vi "Camera.vi"(0 "Camera in":refnum<class "Camera.lvclass">, 1 "Stop":bool, 4 "BCG Image Processing":T3={"Brightness"=128.0, "Contrast"=45.0, "Gamma"=1.0} {"Brightness" scale=0.0..400.0; "Contrast" scale=0.0..90.0; "Gamma" scale=0.005..5.0}, 5 "error in (no error)":errorcluster, 6 "Machine Vision":T5, 7 "Camera settings":T2={"Gamma"=1.0, "Gain"=7, "Sharpness"=0, "Contrast"=0.009999999999999995, "Exposure"=0.0004073180282999787} {"Exposure" min=0.000244140625 max=0.5 scale=0.0002..0.5; "Contrast" min=0.0 max=1.0 scale=0.001..1.0; "Sharpness" min=0 max=2 step=1 scale=0.0..2.0; "Gain" min=0 max=100 step=1 scale=0.1..100.0; "Gamma" min=0.01 max=10.0 scale=0.01..10.0}, 10 "Material":T4, 12 "Loop 0":bool, 13 "Override presets":bool) -> (11 "Radius (Real-World)":dbl, 14 "Camera out":refnum<class "Camera.lvclass">, 15 "Average Strength":dbl, 16 "Global Report":T1 {"Mean Value" format="%.2f"; "%" format="%.2f"; "Area (calibrated)" format="%.2f"; "Maximal Value" format="%.2f"; "Minimal Value" format="%.2f"; "Standard Variation" format="%.2f"}, 17 "Image":T6(plugin-control), 18 "Camera":dbl[](array[numeric]), 19 "error out":errorcluster)   [LabVIEW 2021, in "Camera.lvclass"]
uses:
  Camera.lvclass
  Machine Vision.ctl
  Material.ctl
  Image processing.ctl
  Camera settings.ctl
  <vilib>/vision/NI_Vision_Development_Module.lvlib
panel:
  out "Y":sgl
  out "X":sgl
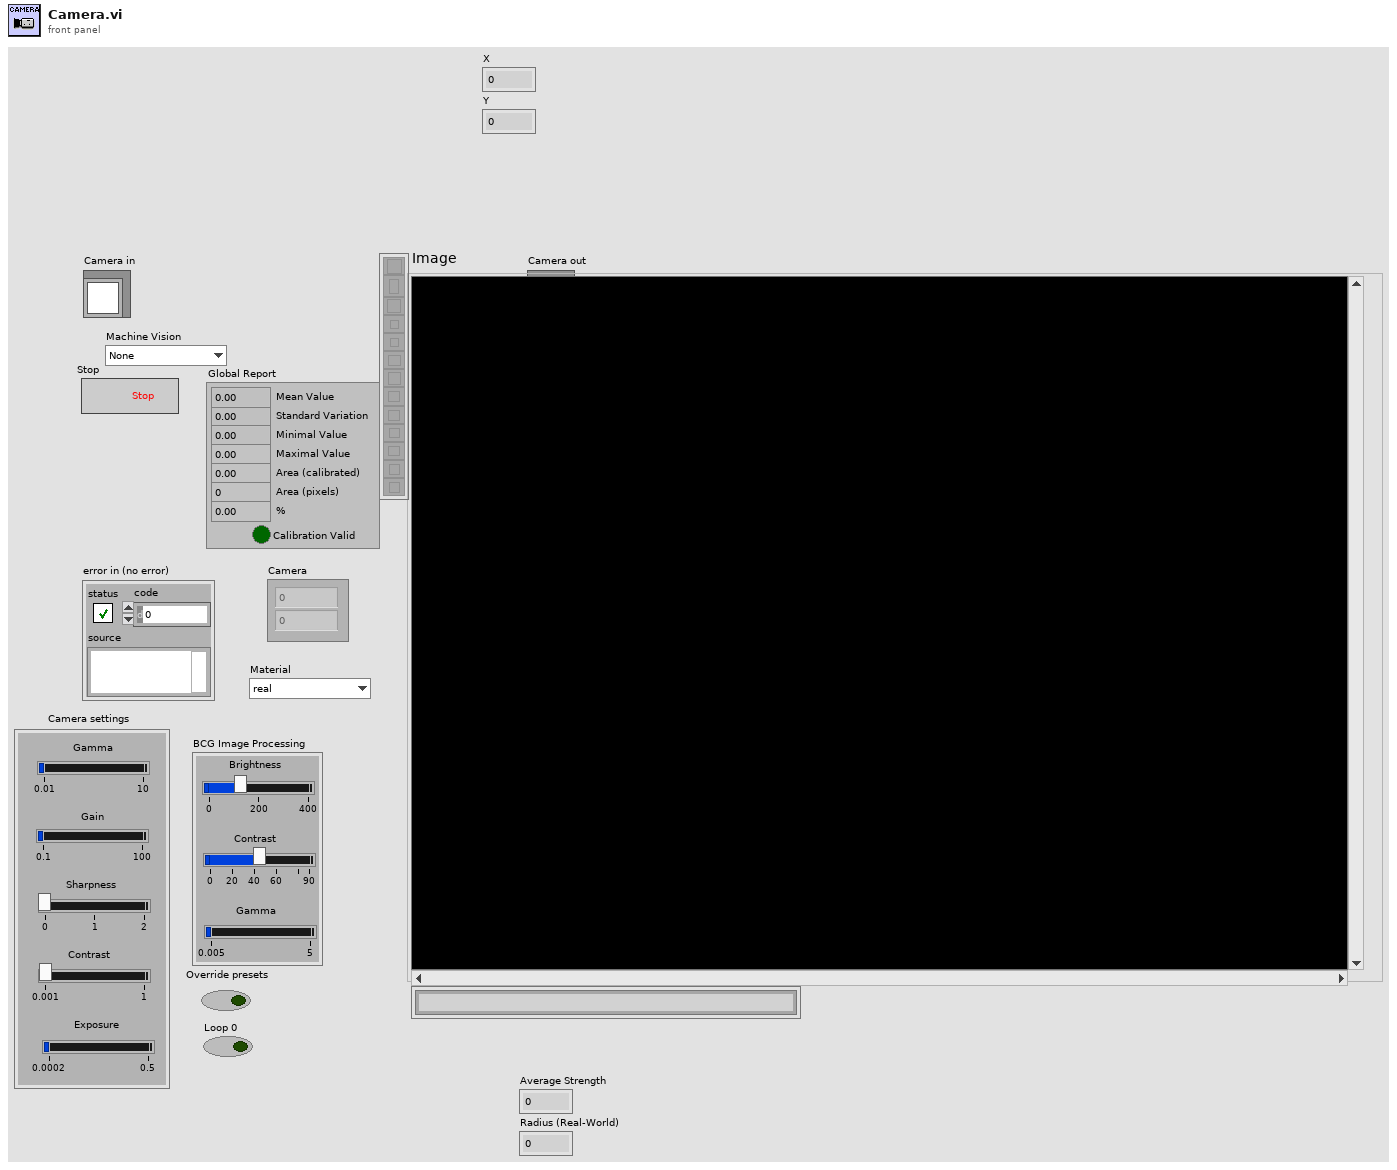
[diagram p1: front panel]
types:
  T1 = cluster{"Mean Value":sgl, "Standard Variation":sgl, "Minimal Value":sgl, "Maximal Value":sgl, "Area (calibrated)":sgl, "Area (pixels)":u32, "%":sgl, "Calibration Valid":bool}
  T2 = typedef "Camera.lvclass/Camera settings.ctl" = cluster{"Gamma":dbl, "Gain":i64, "Sharpness":i64, "Contrast":dbl, "Exposure":dbl}
  T3 = typedef "Camera.lvclass/Image processing.ctl" = cluster{"Brightness":sgl, "Contrast":sgl, "Gamma":sgl}
  T4 = typedef "Camera.lvclass/Material.ctl" = enum16{"real", "dummy", "PETG"}
  T5 = typedef "Camera.lvclass/Machine Vision.ctl" = enum16{"None", "Tray Fiducials", "Sensor Fiducials", "HPK Silicon", "Partial Hexaboard", "Partial Hexaboard Test", "100um dot", "Hexaboard", "Corner (TL, BR)", "Corner (BL, TR)", "V3 Sensor Cross", "V3 Sensor Circle"}
  T6 = typedef "IMAQ Image.ctl" = refnum<image>
  T7 = cluster{"Center (Pixels)":cluster{"X":sgl, "Y":sgl}, "Radius (Pixels)":dbl, "Center (Real-World)":cluster{"X":sgl, "Y":sgl}, "Radius (Real-World)":dbl, "Roundness (Real-World)":dbl, "Average Strength":dbl, "Average SNR (dB)":dbl}
  T8 = typedef "Edge New.ctl" = cluster{"Location (Pixel)":cluster{"X":sgl, "Y":sgl}, "Location (Real-World)":cluster{"X":sgl, "Y":sgl}, "Distance (Pixel)":dbl, "Distance (Real-World)":dbl, "Strength":dbl, "Noise":dbl, "Rising?":bool}
  T9 = cluster{"output string":sgl, "output string":sgl}
  T10 = typedef "ROI Descriptor" = cluster{"Global Rectangle":i32[], "Contours":cluster{"ID":enum32{"External", "Internal"}, "Type":u32, "Coordinates":i32[]}[]}
  T11 = typedef "Image Type" = u32
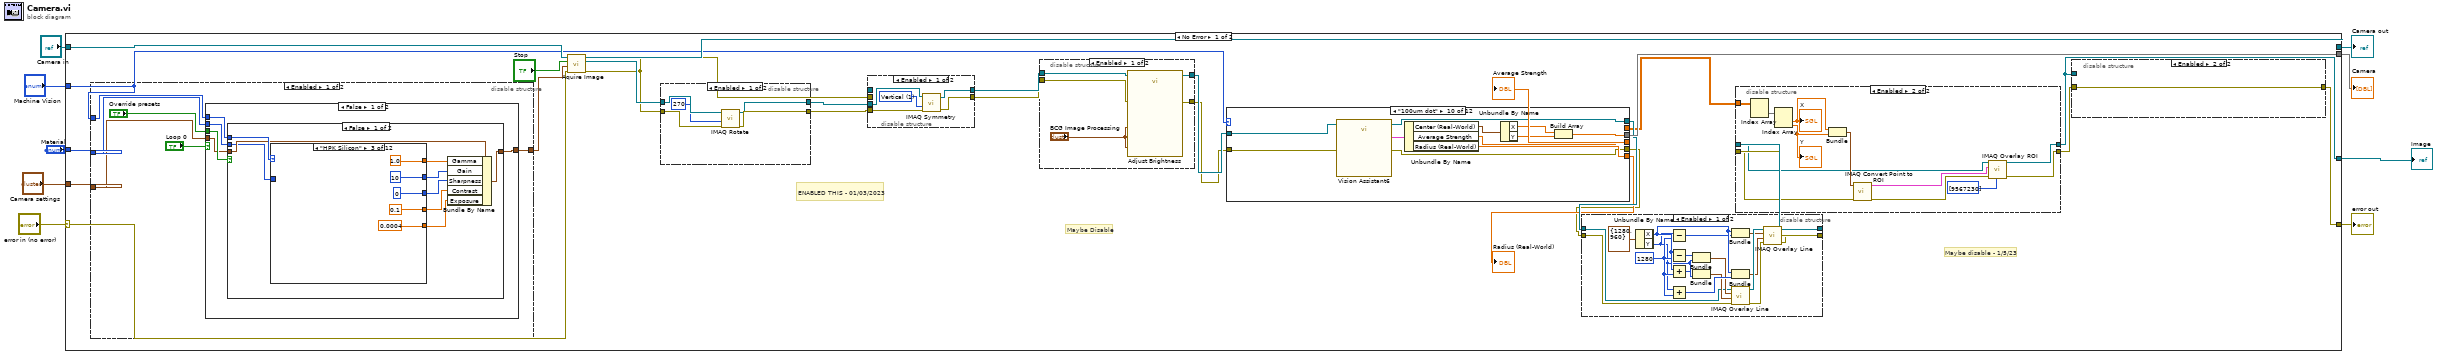
[diagram p0: block diagram]
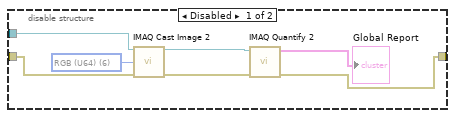
[diagram p2: hidden frame]
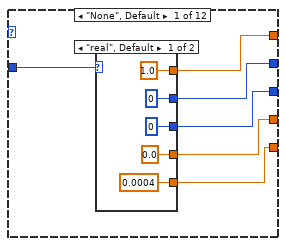
[diagram p7: hidden frame]
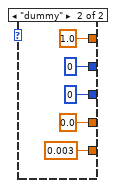
[diagram p8: hidden frame]
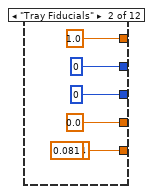
[diagram p9: hidden frame]
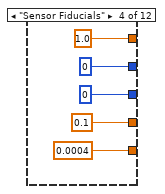
[diagram p10: hidden frame]
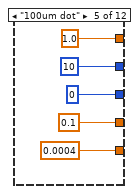
[diagram p11: hidden frame]
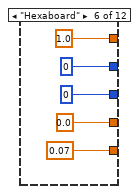
[diagram p12: hidden frame]
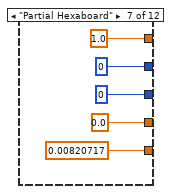
[diagram p13: hidden frame]
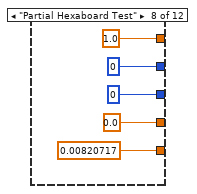
[diagram p14: hidden frame]
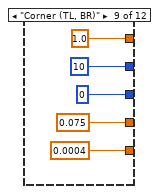
[diagram p15: hidden frame]
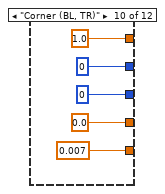
[diagram p16: hidden frame]
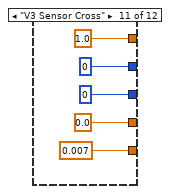
[diagram p17: hidden frame]
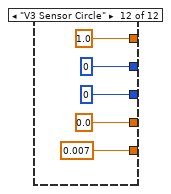
[diagram p18: hidden frame]
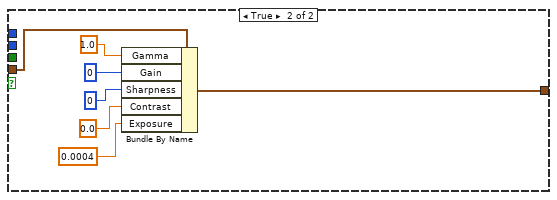
[diagram p20: hidden frame]
diagram:
  n1 = case shown="No Error" "error in (no error)" {
    selector: "error in (no error)" -> [w20 w327]
    tunnel: [w10 w327] -> w8
    tunnel: [w34 w326] -> w7
    tunnel: "Camera in" -> [w35 w326]
    tunnel: [w33 _] -> w5
    tunnel: [w12 _] -> w4
    tunnel: "Machine Vision" -> [w29 _]
    tunnel: "Camera settings" -> [w30 _]
    tunnel: "Material" -> [w28 _]
    frame No Error {
      # "Maybe Disable"
      # "Maybe disable - 1/5/23"
      # "ENABLED THIS - 01/03/2023"
      n2 = disable-structure shown="Enabled" {
        disable-tunnel: w29 -> [w98 _]
        disable-tunnel: w30 -> [w97 w192]
        disable-tunnel: [w96 w192] -> w31
        disable-tunnel: w28 -> [w93 _]
        frame Enabled {
          n3 = case shown="False" "Loop 0" {
            tunnel: "Override presets" -> [w103 _]
            tunnel: w98 -> [w102 _]
            tunnel: w97 -> [w101 w191]
            tunnel: [w100 w190] -> w96
            tunnel: w93 -> [w99 _]
            frame False {
              n4 = case shown="False" w103 {
                tunnel: w102 -> [w112 _]
                tunnel: w101 -> [w111 w184]
                tunnel: [w105 w184] -> w100
                tunnel: w99 -> [w104 _]
                frame False {
                  n5 = case shown="\"HPK Silicon\"" w112 {
                    tunnel: [w117 1.0 ("Gamma::Value") 1.0 ("Gamma::Value") 1.0 ("Gamma::Value") 1.0 ("Gamma::Value") 1.0 ("Gamma::Value") 1.0 ("Gamma::Value") 1.0 ("Gamma::Value") 1.0 ("Gamma::Value") 1.0 ("Gamma::Value") 1.0 ("Gamma::Value") 1.0 ("Gamma::Value")] -> w110
                    tunnel: [w113 i64 0 ("Gain::Value") i64 10 ("Gain::Value") i64 0 ("Gain::Value") i64 10 ("Gain::Value") i64 0 ("Gain::Value") i64 0 ("Gain::Value") i64 0 ("Gain::Value") i64 10 ("Gain::Value") i64 0 ("Gain::Value") i64 0 ("Gain::Value") i64 0 ("Gain::Value")] -> w109
                    tunnel: [w114 i64 0 ("Sharpness::Value") i64 0 ("Sharpness::Value") i64 0 ("Sharpness::Value") i64 0 ("Sharpness::Value") i64 0 ("Sharpness::Value") i64 0 ("Sharpness::Value") i64 0 ("Sharpness::Value") i64 0 ("Sharpness::Value") i64 0 ("Sharpness::Value") i64 0 ("Sharpness::Value") i64 0 ("Sharpness::Value")] -> w108
                    tunnel: [w115 0.0 ("Contrast::Value") 0.1 ("Contrast::Value") 0.1 ("Contrast::Value") 0.1 ("Contrast::Value") 0.0 ("Contrast::Value") 0.0 ("Contrast::Value") 0.0 ("Contrast::Value") 0.075 ("Contrast::Value") 0.0 ("Contrast::Value") 0.0 ("Contrast::Value") 0.0 ("Contrast::Value")] -> w107
                    tunnel: [w116 0.081 ("Exposure::Value") 0.0004 ("Exposure::Value") 0.0004 ("Exposure::Value") 0.0004 ("Exposure::Value") 0.07 ("Exposure::Value") 0.00820717 ("Exposure::Value") 0.00820717 ("Exposure::Value") 0.0004 ("Exposure::Value") 0.007 ("Exposure::Value") 0.007 ("Exposure::Value") 0.007 ("Exposure::Value")] -> w106
                    tunnel: w104 -> [w118 _ _ _ _ _ _ _ _ _ _ _]
                    frame "None", Default {
                      n6 = case shown="\"real\", Default" w118 {
                        tunnel: [1.0 ("Gamma::Value") 1.0 ("Gamma::Value")] -> w117
                        tunnel: [0.0004 ("Exposure::Value") 0.003 ("Exposure::Value")] -> w116
                        tunnel: [0.0 ("Contrast::Value") 0.0 ("Contrast::Value")] -> w115
                        tunnel: [i64 0 ("Sharpness::Value") i64 0 ("Sharpness::Value")] -> w114
                        tunnel: [i64 0 ("Gain::Value") i64 0 ("Gain::Value")] -> w113
                        frame "real", Default {
                        }
                        frame "dummy" {
                        }
                      }
                    }
                    frame "Tray Fiducials" {
                      (unwired) 0.0004 ("Exposure::Value")
                    }
                    frame "HPK Silicon" {
                    }
                    frame "Sensor Fiducials" {
                    }
                    frame "100um dot" {
                    }
                    frame "Hexaboard" {
                    }
                    frame "Partial Hexaboard" {
                    }
                    frame "Partial Hexaboard Test" {
                    }
                    frame "Corner (TL, BR)" {
                    }
                    frame "Corner (BL, TR)" {
                    }
                    frame "V3 Sensor Cross" {
                    }
                    frame "V3 Sensor Circle" {
                    }
                  }
                  n7 = Bundle By Name(cluster=w111, "Gamma"=w110, "Gain"=w109, "Sharpness"=w108, "Contrast"=w107, "Exposure"=w106) -> (w105:T2)
                }
                frame True {
                }
              }
            }
            frame True {
              n8 = Bundle By Name(cluster=w191, "Gamma"=1.0, "Gain"=i64 0, "Sharpness"=i64 0, "Contrast"=0.0, "Exposure"=0.0004) -> (w190:T2)
            }
          }
        }
        frame Disabled {
        }
      }
      n9 = call-dynamic "Aquire Image.vi"("error in (no error)"=w20, "Cluster"=w31, "Stop"="Stop", "Camera in"=w35) -> ("error out"=w19:errorcluster, "Image Out"=w32:T6, "Camera out"=w34:refnum<class "Camera.lvclass">)  [unwired: 5 in]
      n10 = disable-structure shown="Enabled" {
        disable-tunnel: w32 -> [w49 w51]
        disable-tunnel: w19 -> [w48 w50]
        disable-tunnel: [w46 w50] -> w14
        disable-tunnel: [w45 w51] -> w13
        frame Enabled {
          n11 = call "IMAQ Rotate"("error in (no error)"=w48, "Angle (degrees)"=270, "Image Src"=w49) -> ("error out"=w46:errorcluster, "Image Dst Out"=w45:T6)  [unwired: 7 in]
        }
        frame Disabled {
        }
      }
      n12 = disable-structure shown="Enabled" {
        disable-tunnel: _ -> [_ w199]
        disable-tunnel: [w197 w199] -> w27
        disable-tunnel: w19 -> [_ w198]
        disable-tunnel: [w195 w198] -> w18
        disable-tunnel: w14 -> [w194 _]
        disable-tunnel: w13 -> [w193 _]
        frame Enabled {
          w196 = u32 1 items=["Horizontal", "Vertical", "Central", "1st Diagonal", "2nd Diagonal"] ("Type of Symmetry")
          n13 = call "IMAQ Symmetry"("error in (no error)"=w194, "Type of Symmetry"=w196, "Image Src"=w193) -> ("error out"=w195:errorcluster, "Image Dst Out"=w197:T6)  [unwired: 2 in]
        }
        frame Disabled {
        }
      }
      n14 = disable-structure shown="Enabled" {
        disable-tunnel: w27 -> [w90 w91]
        disable-tunnel: [w88 w91] -> w26
        disable-tunnel: w18 -> [w87 w92]
        disable-tunnel: [w86 w92] -> w17
        frame Enabled {
          n15 = call "Adjust Brightness"("Image In"=w90, "Red BCG Values (Brightness 1)"="BCG Image Processing", "Green BCG Values (Brightness 1)"="BCG Image Processing", "Blue BCG Values (Brightness 1)"="BCG Image Processing", "error in"=w87) -> ("Image Out"=w88:T6, "error out"=w86:errorcluster)  [unwired: 21 in]
        }
        frame Disabled {
        }
      }
      n16 = case shown="\"100um dot\"" w29 {
        tunnel: [w204 w214 w222 w233 w244 w255 w266 w275 w286 w297 w303 w315] -> w33
        tunnel: [w206 w216 w223 w234 w245 w256 w268 w276 w287 w298 w307 w319] -> w25
        tunnel: w26 -> [w207 w216 w221 w232 w243 w254 w265 w273 w284 w295 w308 w320]
        tunnel: [w202 0.0 ("Radius (Real-World)") w219 w230 w241 w252 0.0 ("Radius (Real-World)") w272 w283 w294 0.0 ("Radius (Real-World)") 0.0 ("Radius (Real-World)")] -> w23
        tunnel: [w203 0.0 ("Strength") w220 w231 w242 w253 _ w271 w282 w293 w313 w325] -> w22
        tunnel: [_ _ _ _ _ _ w264 _ _ _ _ _] -> w21
        tunnel: w17 -> [w201 w215 w217 w228 w239 w250 w263 w270 w281 w292 w306 w318]
        tunnel: [w200 w215 w218 w229 w240 w251 w262 w269 w280 w291 w305 w317] -> w16
        frame "Tray Fiducials", Default {
          n17 = call "Vision Assistant"("Image In"=w207, "error in"=w201) -> ("Image Out"=w206:T6, "Fitted Circle (Find Circular Edge 1)"=w205:T7, "error out"=w200:errorcluster)  [unwired: 23 in]
          n18 = Unbundle By Name(w205) -> ("Center (Real-World)"=w208:cluster{"X":sgl, "Y":sgl}, "Average Strength"=w203:dbl, "Radius (Real-World)"=w202:dbl)
          n19 = Unbundle By Name(w208) -> ("X"=w210:sgl, "Y"=w209:sgl)
          n20 = Build Array(w210, w209) -> (w204:sgl[])
        }
        frame "None" {
          n21 = Initialize Array(0.0 ("element")) -> (w214:dbl[])  [unwired: 1 in]
        }
        frame "Hexaboard" {
          n22 = call "Vision Assistant2"("Image In"=w221, "error in"=w217) -> ("Image Out"=w223:T6, "Fitted Circle (Find Circular Edge 1)"=w225:T7, "error out"=w218:errorcluster)  [unwired: 23 in]
          n23 = Unbundle By Name(w225) -> ("Center (Real-World)"=w227:cluster{"X":sgl, "Y":sgl}, "Average Strength"=w220:dbl, "Radius (Real-World)"=w219:dbl)
          n24 = Unbundle By Name(w227) -> ("X"=w226:sgl, "Y"=w224:sgl)
          n25 = Build Array(w226, w224) -> (w222:sgl[])
        }
        frame "V3 Sensor Circle" {
          n26 = call "Vision Assistant4"("Image In"=w232, "error in"=w228) -> ("Image Out"=w234:T6, "Fitted Circle (Find Circular Edge 1)"=w236:T7, "error out"=w229:errorcluster)  [unwired: 23 in]
          n27 = Unbundle By Name(w236) -> ("Center (Real-World)"=w238:cluster{"X":sgl, "Y":sgl}, "Average Strength"=w231:dbl, "Radius (Real-World)"=w230:dbl)
          n28 = Unbundle By Name(w238) -> ("X"=w237:sgl, "Y"=w235:sgl)
          n29 = Build Array(w237, w235) -> (w233:sgl[])
        }
        frame "Partial Hexaboard" {
          n30 = call "Vision Assistant20"("Image In"=w243, "error in"=w239) -> ("Image Out"=w245:T6, "Fitted Circle (Find Circular Edge 1)"=w247:T7, "error out"=w240:errorcluster)  [unwired: 23 in]
          n31 = Unbundle By Name(w247) -> ("Center (Real-World)"=w249:cluster{"X":sgl, "Y":sgl}, "Average Strength"=w242:dbl, "Radius (Real-World)"=w241:dbl)
          n32 = Unbundle By Name(w249) -> ("X"=w248:sgl, "Y"=w246:sgl)
          n33 = Build Array(w248, w246) -> (w244:sgl[])
        }
        frame "Partial Hexaboard Test" {
          n34 = call "Vision Assistant10"("Image In"=w254, "error in"=w250) -> ("Image Out"=w256:T6, "Fitted Circle (Find Circular Edge 1)"=w258:T7, "error out"=w251:errorcluster)  [unwired: 23 in]
          n35 = Unbundle By Name(w258) -> ("Center (Real-World)"=w260:cluster{"X":sgl, "Y":sgl}, "Average Strength"=w253:dbl, "Radius (Real-World)"=w252:dbl)
          n36 = Unbundle By Name(w260) -> ("X"=w259:sgl, "Y"=w257:sgl)
          n37 = Build Array(w259, w257) -> (w255:sgl[])
        }
        frame "Corner (TL, BR)" {
          n38 = call "Vision Assistant3"("Image In"=w265, "error in"=w263) -> ("Image Out"=w268:T6, "error out"=w262:errorcluster, "Caliper Results (Top Left, Bottom Right)"=w264:sgl[][], "Calibrated Results (Top Left, Bottom Right)"=w267:sgl[][])  [unwired: 22 in]
          n39 = Index Array(array=w267) -> (element=w266:sgl[])  [unwired: 2 in]
        }
        frame "HPK Silicon" {
          n40 = call "Vision Assistant5"("Image In"=w273, "error in"=w270) -> ("Image Out"=w276:T6, "Fitted Circle (Find Circular Edge 1)"=w274:T7, "error out"=w269:errorcluster)  [unwired: 23 in]
          n41 = Unbundle By Name(w274) -> ("Center (Real-World)"=w279:cluster{"X":sgl, "Y":sgl}, "Average Strength"=w271:dbl, "Radius (Real-World)"=w272:dbl)
          n42 = Unbundle By Name(w279) -> ("X"=w278:sgl, "Y"=w277:sgl)
          n43 = Build Array(w278, w277) -> (w275:sgl[])
        }
        frame "Sensor Fiducials" {
          n44 = call "Vision Assistant9"("Image In"=w284, "error in"=w281) -> ("Image Out"=w287:T6, "Fitted Circle (Find Circular Edge 1)"=w285:T7, "error out"=w280:errorcluster)  [unwired: 23 in]
          n45 = Unbundle By Name(w285) -> ("Center (Real-World)"=w290:cluster{"X":sgl, "Y":sgl}, "Average Strength"=w282:dbl, "Radius (Real-World)"=w283:dbl)
          n46 = Unbundle By Name(w290) -> ("X"=w289:sgl, "Y"=w288:sgl)
          n47 = Build Array(w289, w288) -> (w286:sgl[])
        }
        frame "100um dot" {
          n48 = call "Vision Assistant6"("Image In"=w295, "error in"=w292) -> ("Image Out"=w298:T6, "Fitted Circle (Find Circular Edge 1)"=w296:T7, "error out"=w291:errorcluster)  [unwired: 23 in]
          n49 = Unbundle By Name(w296) -> ("Center (Real-World)"=w301:cluster{"X":sgl, "Y":sgl}, "Average Strength"=w293:dbl, "Radius (Real-World)"=w294:dbl)
          n50 = Unbundle By Name(w301) -> ("X"=w300:sgl, "Y"=w299:sgl)
          n51 = Build Array(w300, w299) -> (w297:sgl[])
        }
        frame "Corner (BL, TR)" {
          n52 = call "Vision Assistant7"("Image In"=w308, "error in"=w306) -> ("Image Out"=w307:T6, "Used Edges (Adv. Straight Edge 1)"=w312:cluster{"Edge Information":T8[]}[], "error out"=w305:errorcluster)  [unwired: 23 in]
          n53 = Index Array(array=w312) -> (element=w311:cluster{"Edge Information":T8[]})  [unwired: 1 in]
          n54 = Unbundle By Name(w311) -> ("Edge Information"=w310:T8[])
          n55 = Index Array(array=w310) -> (element=w309:T8)  [unwired: 1 in]
          n56 = Unbundle(w309) -> ("Location (Real-World)"=w304:cluster{"X":sgl, "Y":sgl}, "Strength"=w313:dbl)  [unwired: 5 out]
          n57 = Cluster To Array(cluster=w304) -> (array=w303:sgl[])
        }
        frame "V3 Sensor Cross" {
          n58 = call "Vision Assistant8"("Image In"=w320, "error in"=w318) -> ("Image Out"=w319:T6, "Used Edges (Adv. Straight Edge 1)"=w324:cluster{"Edge Information":T8[]}[], "error out"=w317:errorcluster)  [unwired: 23 in]
          n59 = Index Array(array=w324) -> (element=w323:cluster{"Edge Information":T8[]})  [unwired: 1 in]
          n60 = Unbundle By Name(w323) -> ("Edge Information"=w322:T8[])
          n61 = Index Array(array=w322) -> (element=w321:T8)  [unwired: 1 in]
          n62 = Unbundle(w321) -> ("Location (Real-World)"=w316:cluster{"X":sgl, "Y":sgl}, "Strength"=w325:dbl)  [unwired: 5 out]
          n63 = Cluster To Array(cluster=w316) -> (array=w315:sgl[])
        }
      }
      "Radius (Real-World)" <- w23
      "Average Strength" <- w22
      n64 = disable-structure shown="Enabled" {
        disable-tunnel: w25 -> [w70 w85]
        disable-tunnel: [w69 w85] -> w24
        disable-tunnel: w16 -> [w68 w84]
        disable-tunnel: [w66 w84] -> w15
        frame Enabled {
          w77 = 1280
          n65 = Unbundle By Name(cluster{"X":i32, "Y":i32} {"X"=1280, "Y"=960} ("Cross Hair coordinates")) -> ("X"=w80:i32, "Y"=w76:i32)
          n66 = Subtract(x=w76, y=w77) -> (x-y=w78:i32)
          n67 = Subtract(x=w80, y=w77) -> (x-y=w72:i32)
          n68 = Add(x=w80, y=w77) -> (x+y=w73:i32)
          n69 = Add(x=w76, y=w77) -> (x+y=w79:i32)
          n70 = Bundle(w72, "Y"=w76) -> (w75:cluster{i32, "Y":i32})  [unwired: 1 in]
          n71 = Bundle(w73, "Y"=w76) -> (w74:cluster{i32, "Y":i32})  [unwired: 1 in]
          n72 = Bundle("X"=w80, w78) -> (w81:cluster{"X":i32, i32})  [unwired: 1 in]
          n73 = Bundle("X"=w80, w79) -> (w82:cluster{"X":i32, i32})  [unwired: 1 in]
          n74 = call "IMAQ Overlay Line"("error in (no error)"=w68, "End Point"=w74, "Start Point"=w75, "Image"=w70) -> ("error out"=w67:errorcluster, "Image Out"=w83:T6)  [unwired: 6 in]
          n75 = call "IMAQ Overlay Line"("error in (no error)"=w67, "End Point"=w82, "Start Point"=w81, "Image"=w83) -> ("error out"=w66:errorcluster, "Image Out"=w69:T6)  [unwired: 6 in]
        }
        frame Disabled {
        }
      }
      n76 = disable-structure shown="Enabled" {
        disable-tunnel: [w53 w61] -> w12
        disable-tunnel: w24 -> [w53 w60]
        disable-tunnel: w21 -> [_ w59]
        disable-tunnel: w15 -> [w52 w56]
        disable-tunnel: [w52 w54] -> w11
        frame Disabled {
        }
        frame Enabled {
          n77 = Index Array(array=w59) -> (element=w58:sgl[])  [unwired: 2 in]
          n78 = Index Array(array=w58) -> (element #1=w62:sgl, element #2=w64:sgl)  [unwired: 2 in]
          "X" <- w62
          "Y" <- w64
          n79 = Bundle("output string"=w62, "output string"=w64) -> (w65:T9)  [unwired: 1 in]
          n80 = call "IMAQ Convert Point to ROI"("error in (no error)"=w56, "Point"=w65) -> ("error out"=w55:errorcluster, "ROI Descriptor"=w63:T10)  [unwired: 7 in]
          n81 = call "IMAQ Overlay ROI"("Colors (Green)"=u32[] [9567230], "error in (no error)"=w55, "ROI Descriptor"=w63, "Image"=w60) -> ("error out"=w54:errorcluster, "Image Out"=w61:T6)  [unwired: 6 in]
        }
      }
      n82 = disable-structure shown="Enabled" {
        disable-tunnel: w12 -> [w39 _]
        disable-tunnel: w11 -> [w41 w44]
        disable-tunnel: [w42 w44] -> w10
        frame Disabled {
          w38 = T11 6 items=["Grayscale (U8)", "Grayscale (I16)", "Grayscale (SGL)", "Complex (CSG)", "RGB (U32)", "HSL (U32)", "RGB (U64)", "Grayscale (U16)"] ("Image Type")
          n83 = call "IMAQ Cast Image 2"("Image Src"=w39, "Image Type"=w38, "error in (no error)"=w41) -> ("Image Dst Out"=w37:T6, "error out"=w40:errorcluster)  [unwired: 11 in]
          n84 = call "IMAQ Quantify 2"("error in (no error)"=w40, "Image"=w37) -> ("error out"=w42:errorcluster, "Global Report"=→"Global Report":T1)  [unwired: 7 in, 1 out]
        }
        frame Enabled {
        }
      }
    }
    frame Error {
    }
  }
  "error out" <- w8
  "Camera out" <- w7
  "Camera" <- w5
  "Image" <- w4
